vi "Handle Value Change - Add to Owner.vi"(8 "Error In":errorcluster, 10 "New Value":bool, 11 "Module Data In":T1) -> (0 "Error Out":errorcluster)   [LabVIEW 2022 SP3]
doc: "This VI handles the Value Change event on the \"Add To Owner?\" checkbox.\n\nAcronyms\nATP = \"Add To Project?\" checkbox\nATO = \"Add To Owner?\" checkbox\nATVF = \"Add To Virtual Folder?\" checkbox"
uses:
  Module Data.ctl
  GUI Object Refs (cluster).ctl
  Initial State (enum).ctl
  Input Conditions (cluster).ctl
  DFS Output (cluster).ctl
panel:
  # "Development\nControls or indicators that are useful for development or testing, but which are not outputs of the VI."
  # "Input\nInputs to the VI"
  # "Output\nOutputs of the VI"
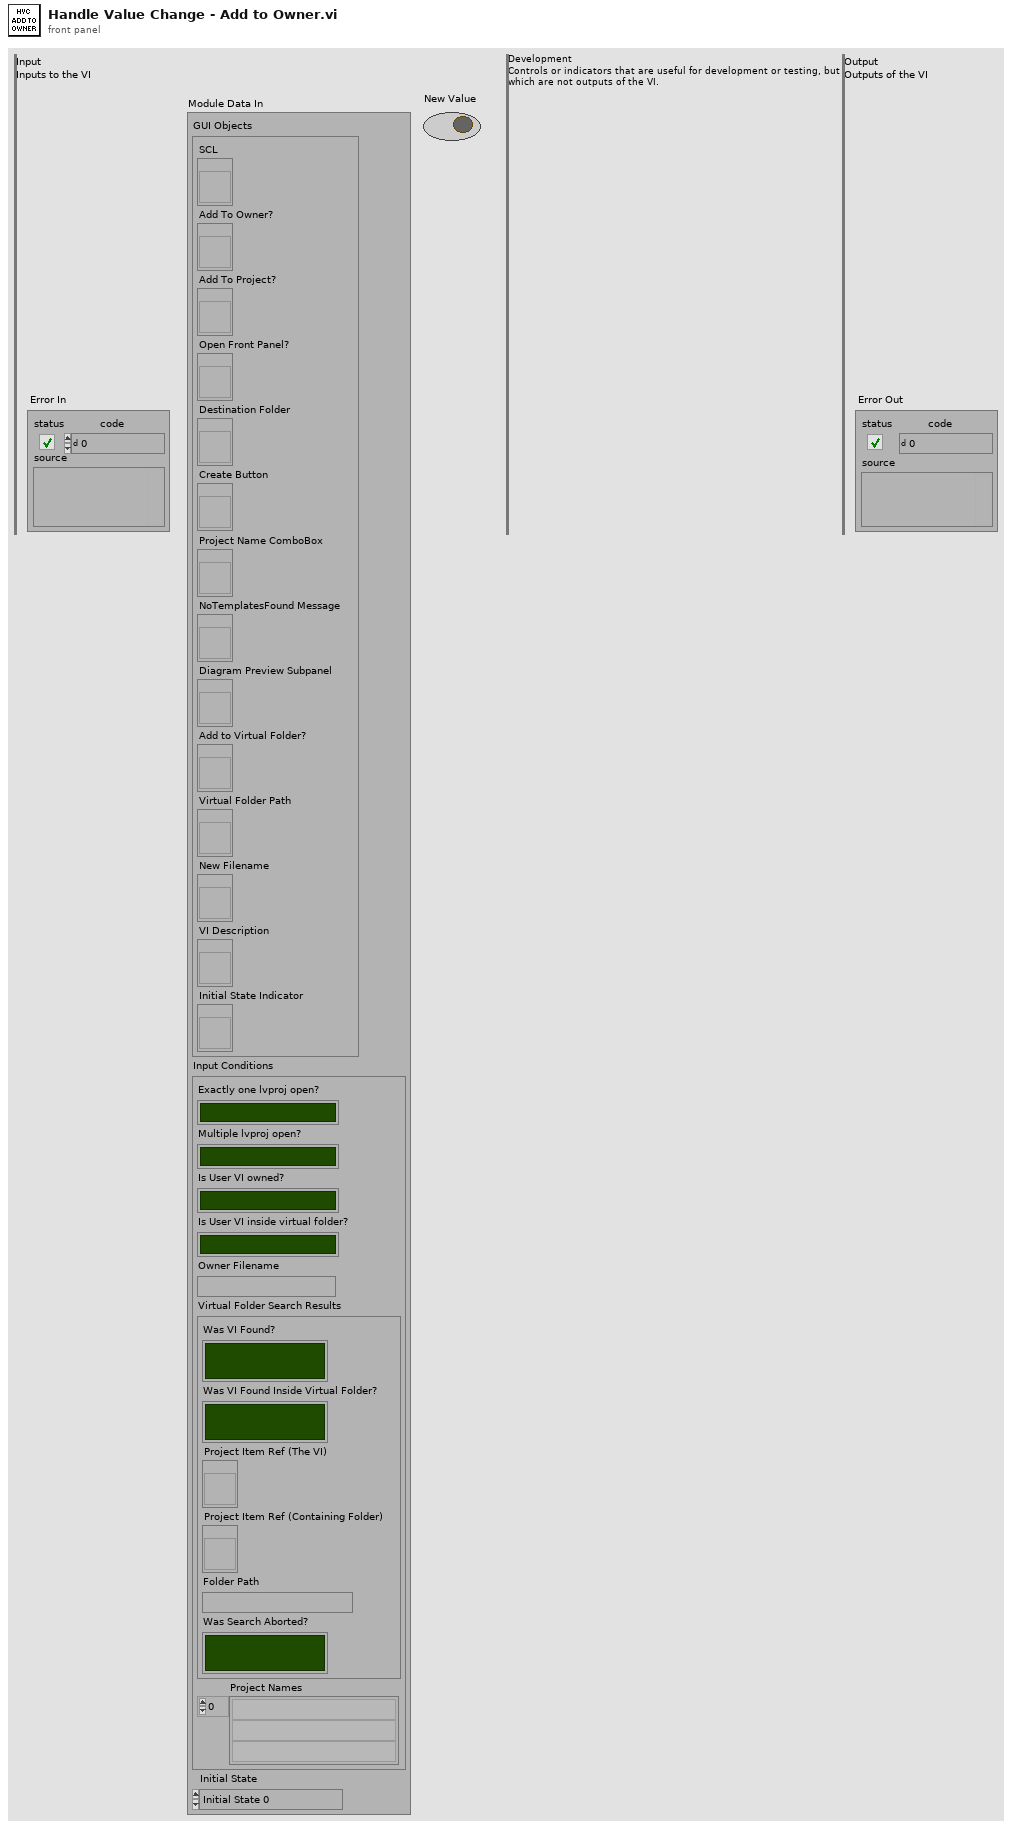
[diagram p1: front panel]
types:
  T1 = typedef "Module Data.ctl" = cluster{"GUI Objects":T2, "Input Conditions":T3, "Initial State":T5}
  T2 = typedef "GUI Object Refs (cluster).ctl" = cluster{"SCL":refnum<vi>, "Add To Owner?":refnum<vi>, "Add To Project?":refnum<vi>, "Open Front Panel?":refnum<vi>, "Destination Folder":refnum<vi>, "Create Button":refnum<vi>, "Project Name ComboBox":refnum<vi>, "NoTemplatesFound Message":refnum<vi>, "Diagram Preview Subpanel":refnum<vi>, "Add to Virtual Folder?":refnum<vi>, "Virtual Folder Path":refnum<vi>, "New Filename":refnum<vi>, "VI Description":refnum<vi>, "Initial State Indicator":refnum<vi>}
  T3 = typedef "Input Conditions (cluster).ctl" = cluster{"Exactly one lvproj open?":bool, "Multiple lvproj open?":bool, "Is User VI owned?":bool, "Is User VI inside virtual folder?":bool, "Owner Filename":string, "Virtual Folder Search Results":T4, "Project Names":string[]}
  T4 = typedef "DFS Output (cluster).ctl" = cluster{"Was VI Found?":bool, "Was VI Found Inside Virtual Folder?":bool, "Project Item Ref (The VI)":refnum<vi>, "Project Item Ref (Containing Folder)":refnum<vi>, "Folder Path":string, "Was Search Aborted?":bool}
  T5 = typedef "Initial State (enum).ctl" = enum16{"Initial State 0", "Initial State 1", "Initial State 2", "Initial State 3", "Initial State 4", "Initial State 5", "Initial State 6", "Initial State 7", "Initial State 8", "Initial State 9", "Initial State 10", "Initial State 11", "Initial State 12", "Initial State 13", "Initial State 14", "Initial State 15"}
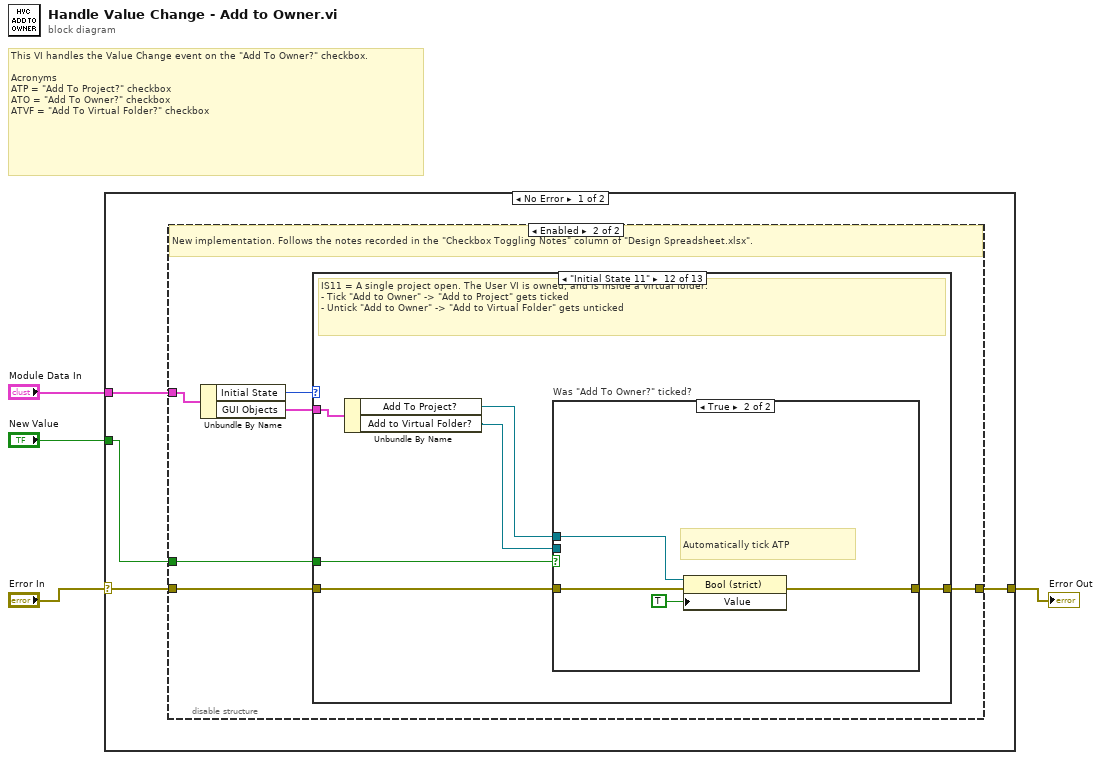
[diagram p0: block diagram]
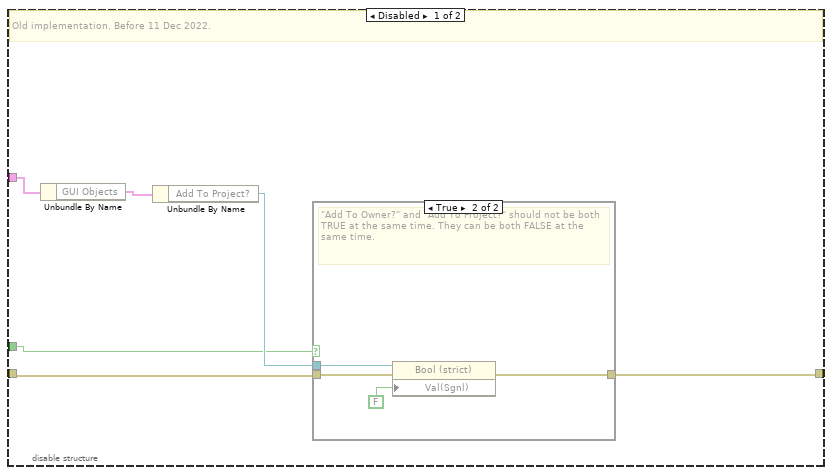
[diagram p2: hidden frame]
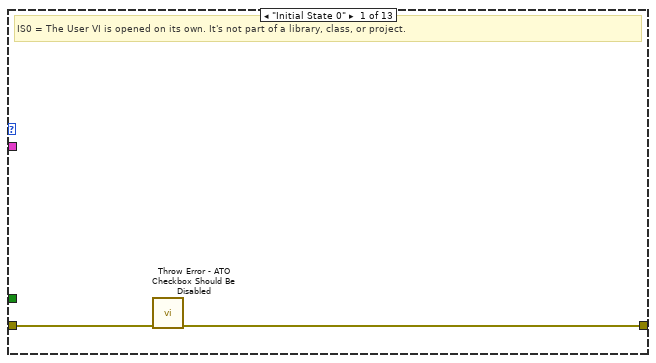
[diagram p4: hidden frame]
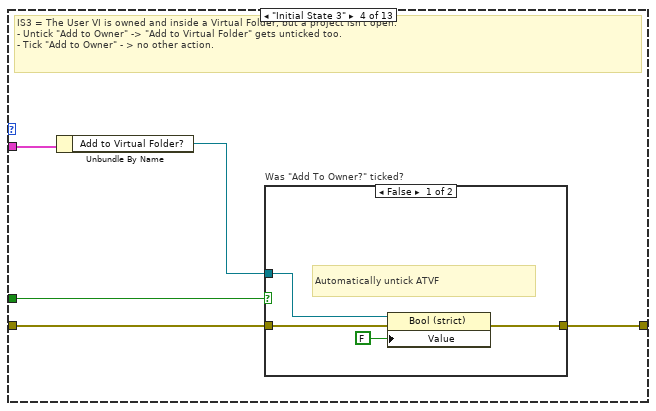
[diagram p7: hidden frame]
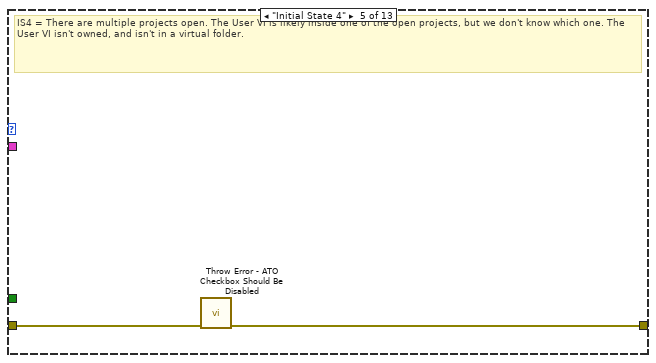
[diagram p9: hidden frame]
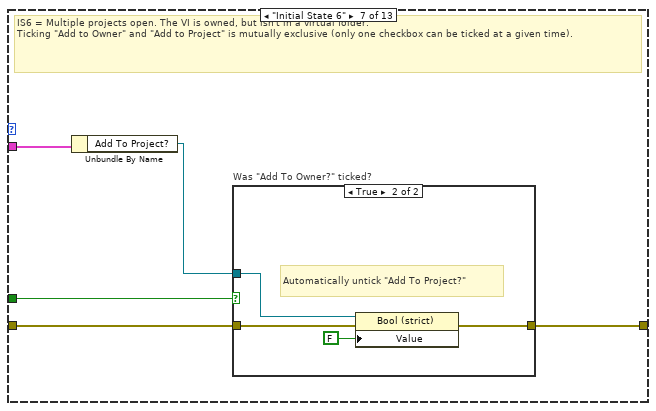
[diagram p11: hidden frame]
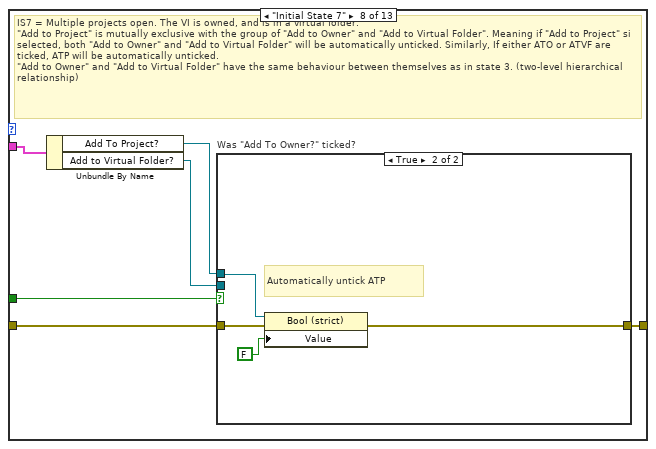
[diagram p13: hidden frame]
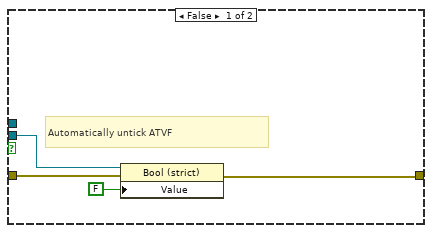
[diagram p14: hidden frame]
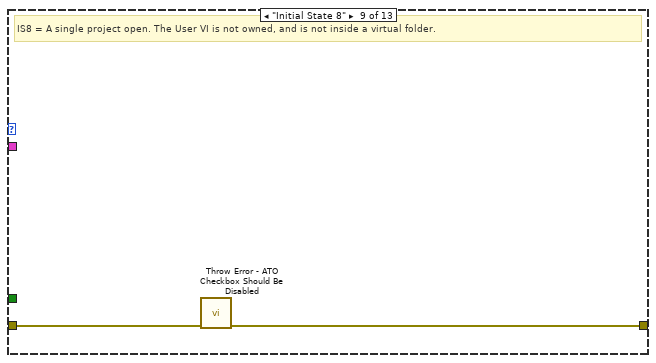
[diagram p15: hidden frame]
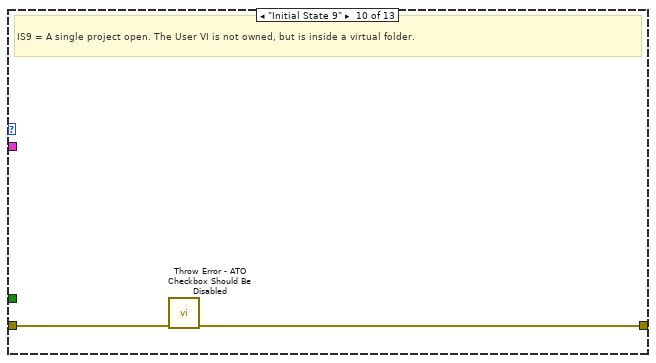
[diagram p16: hidden frame]
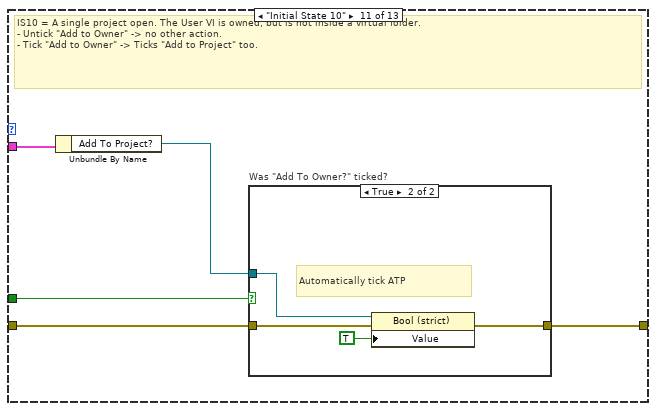
[diagram p17: hidden frame]
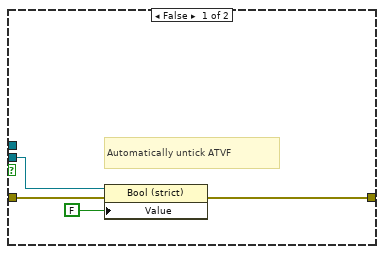
[diagram p19: hidden frame]
diagram:
  # "This VI handles the Value Change event on the \"Add To Owner?\" checkbox.\n\nAcronyms\nATP = \"Add To Project?\" checkbox\nATO = \"Add To Owner?\" checkbox\nATVF = \"Add To Virtual Folder?\" checkbox"
  n1 = case shown="No Error" "Error In" {
    selector: "Error In" -> [w8 w96]
    tunnel: [w7 w96] -> w3
    tunnel: "Module Data In" -> [w6 _]
    tunnel: "New Value" -> [w5 _]
    frame No Error {
      n2 = disable-structure shown="Enabled" {
        disable-tunnel: w8 -> [w12 w25]
        disable-tunnel: [w11 w23] -> w7
        disable-tunnel: w6 -> [w9 w24]
        disable-tunnel: w5 -> [w10 w21]
        frame Disabled {
          # "Old implementation. Before 11 Dec 2022."
          n3 = Unbundle By Name(w9) -> ("GUI Objects"=w14:T2)
          n4 = Unbundle By Name(w14) -> ("Add To Project?"=w13:refnum<vi>)
          n5 = case shown="True" w10 {
            tunnel: w12 -> [w15 w19]
            tunnel: [w15 w18] -> w11
            tunnel: w13 -> [_ w16]
            frame False {
            }
            frame True {
              # "\"Add To Owner?\" and \"Add To Project?\" should not be both TRUE at the same time. They can be both FALSE at the same time."
              n6 = property class="Bool (strict)"(reference=w16, error in=w19, "Val(Sgnl)"=FALSE ("Value (Signaling)")) -> (error out=w18:errorcluster)  [unwired: 1 out]
            }
          }
        }
        frame Enabled {
          # "New implementation. Follows the notes recorded in the \"Checkbox Toggling Notes\" column of \"Design Spreadsheet.xlsx\"."
          n7 = Unbundle By Name(w24) -> ("Initial State"=w22:T5, "GUI Objects"=w20:T2)
          n8 = case shown="\"Initial State 11\"" w22 {
            tunnel: w25 -> [w27 w28 w29 w33 w41 w42 w47 w57 w68 w70 w74 w85 w95]
            tunnel: [w26 w28 w29 w32 w40 w42 w46 w56 w67 w69 w71 w82 w95] -> w23
            tunnel: w21 -> [_ _ _ w31 _ _ w45 w55 _ _ w73 w84 _]
            tunnel: w20 -> [_ _ _ w30 _ _ w44 w54 _ _ w72 w83 _]
            frame "Initial State 0" {
              # "IS0 = The User VI is opened on its own. It's not part of a library, class, or project."
              n9 = call "Throw Error - ATO Checkbox Should Be Disabled.vi"("error in"=w27) -> ("error out"=w26:errorcluster)  [unwired: 10 in]
            }
            frame "Initial State 1" {
              # "Impossible Initial State. Expected to never occur."
            }
            frame "Initial State 2" {
              # "Do nothing. All other checkboxes are disabled, so they can't be ticked or unticked."
              # "IS2 = The User VI is owned by a library or class, but a project isn't open."
            }
            frame "Initial State 3" {
              # "IS3 = The User VI is owned and inside a Virtual Folder, but a project isn't open.\n- Untick \"Add to Owner\" -> \"Add to Virtual Folder\" gets unticked too.\n- Tick \"Add to Owner\" - > no other action."
              n10 = Unbundle By Name(w30) -> ("Add to Virtual Folder?"=w34:refnum<vi>)
              n11 = case "Was \"Add To Owner?\" ticked?" shown="False" w31 {
                tunnel: w33 -> [w38 w39]
                tunnel: [w37 w39] -> w32
                tunnel: w34 -> [w36 _]
                frame False {
                  # "Automatically untick ATVF"
                  n12 = property class="Bool (strict)"(reference=w36, error in=w38, "Value"=FALSE) -> (error out=w37:errorcluster)  [unwired: 1 out]
                }
                frame True {
                  # "Do nothing."
                }
              }
            }
            frame "Initial State 4" {
              # "IS4 = There are multiple projects open. The User VI is likely inside one of the open projects, but we don't know which one. The User VI isn't owned, and isn't in a virtual folder."
              n13 = call "Throw Error - ATO Checkbox Should Be Disabled.vi"("error in"=w41) -> ("error out"=w40:errorcluster)  [unwired: 10 in]
            }
            frame "Initial State 5" {
              # "Impossible Initial State. Expected to never occur."
            }
            frame "Initial State 6" {
              # "IS6 = Multiple projects open. The VI is owned, but isn't in a virtual folder.\nTicking \"Add to Owner\" and \"Add to Project\" is mutually exclusive (only one checkbox can be ticked at a given time)."
              n14 = Unbundle By Name(w44) -> ("Add To Project?"=w43:refnum<vi>)
              n15 = case "Was \"Add To Owner?\" ticked?" shown="True" w45 {
                tunnel: w47 -> [w48 w52]
                tunnel: [w48 w51] -> w46
                tunnel: w43 -> [_ w50]
                frame False {
                  # "Do nothing. Don't automatically tick \"Add To Project?\"."
                }
                frame True {
                  # "Automatically untick \"Add To Project?\""
                  n16 = property class="Bool (strict)"(reference=w50, error in=w52, "Value"=FALSE) -> (error out=w51:errorcluster)  [unwired: 1 out]
                }
              }
            }
            frame "Initial State 7" {
              # "IS7 = Multiple projects open. The VI is owned, and is in a virtual folder.\n\"Add to Project\" is mutually exclusive with the group of \"Add to Owner\" and \"Add to Virtual Folder\". Meaning if \"Add to Project\" si selected, both \"Add to Owner\" and \"Add to Virtual Folder\" will be automatically unticked. Similarly, If either ATO or ATVF are ticked, ATP will be automatically unticked.\n\"Add to Owner\" and \"Add to Virtual Folder\" have the same behaviour between themselves as in state 3. (two-level hierarchical relationship)"
              n17 = Unbundle By Name(w54) -> ("Add To Project?"=w58:refnum<vi>, "Add to Virtual Folder?"=w53:refnum<vi>)
              n18 = case "Was \"Add To Owner?\" ticked?" shown="True" w55 {
                tunnel: [w60 w65] -> w56
                tunnel: w58 -> [_ w63]
                tunnel: w57 -> [w61 w66]
                tunnel: w53 -> [w59 _]
                frame False {
                  # "Automatically untick ATVF"
                  n19 = property class="Bool (strict)"(reference=w59, error in=w61, "Value"=FALSE) -> (error out=w60:errorcluster)  [unwired: 1 out]
                }
                frame True {
                  # "Automatically untick ATP"
                  n20 = property class="Bool (strict)"(reference=w63, error in=w66, "Value"=FALSE) -> (error out=w65:errorcluster)  [unwired: 1 out]
                }
              }
            }
            frame "Initial State 8" {
              # "IS8 = A single project open. The User VI is not owned, and is not inside a virtual folder."
              n21 = call "Throw Error - ATO Checkbox Should Be Disabled.vi"("error in"=w68) -> ("error out"=w67:errorcluster)  [unwired: 10 in]
            }
            frame "Initial State 9" {
              # "IS9 = A single project open. The User VI is not owned, but is inside a virtual folder."
              n22 = call "Throw Error - ATO Checkbox Should Be Disabled.vi"("error in"=w70) -> ("error out"=w69:errorcluster)  [unwired: 10 in]
            }
            frame "Initial State 10" {
              # "IS10 = A single project open. The User VI is owned, but is not inside a virtual folder.\n- Untick \"Add to Owner\" -> no other action.\n- Tick \"Add to Owner\" -> Ticks \"Add to Project\" too."
              n23 = Unbundle By Name(w72) -> ("Add To Project?"=w75:refnum<vi>)
              n24 = case "Was \"Add To Owner?\" ticked?" shown="True" w73 {
                tunnel: w74 -> [w76 w80]
                tunnel: [w76 w79] -> w71
                tunnel: w75 -> [_ w78]
                frame False {
                  # "Do nothing."
                }
                frame True {
                  # "Automatically tick ATP"
                  n25 = property class="Bool (strict)"(reference=w78, error in=w80, "Value"=TRUE) -> (error out=w79:errorcluster)  [unwired: 1 out]
                }
              }
            }
            frame "Initial State 11" {
              # "IS11 = A single project open. The User VI is owned, and is inside a virtual folder.\n- Tick \"Add to Owner\" -> \"Add to Project\" gets ticked\n- Untick \"Add to Owner\" -> \"Add to Virtual Folder\" gets unticked"
              n26 = Unbundle By Name(w83) -> ("Add To Project?"=w86:refnum<vi>, "Add to Virtual Folder?"=w81:refnum<vi>)
              n27 = case "Was \"Add To Owner?\" ticked?" shown="True" w84 {
                tunnel: w85 -> [w90 w94]
                tunnel: [w89 w93] -> w82
                tunnel: w86 -> [_ w92]
                tunnel: w81 -> [w87 _]
                frame False {
                  # "Automatically untick ATVF"
                  n28 = property class="Bool (strict)"(reference=w87, error in=w90, "Value"=FALSE) -> (error out=w89:errorcluster)  [unwired: 1 out]
                }
                frame True {
                  # "Automatically tick ATP"
                  n29 = property class="Bool (strict)"(reference=w92, error in=w94, "Value"=TRUE) -> (error out=w93:errorcluster)  [unwired: 1 out]
                }
              }
            }
            frame "Initial State 12".."Initial State 15" {
              # "Impossible Initial State. Expected to never occur."
            }
          }
        }
      }
    }
    frame Error {
    }
  }
  "Error Out" <- w3
